vi "Control Panel Sensors.vi"(11 "Control Panel Motors":T2) -> (1 "Color":T1, 2 "Arm Out":bool, 3 "Arm In":bool, 4 "Control Panel Full":dbl, 6 "Control Panel":dbl(knob) scale=0.0..1.0, 8 "Arm":dbl(knob) scale=0.0..1.0)   [LabVIEW 2019]
uses:
  Control Panel Motors.ctl
  Color.ctl
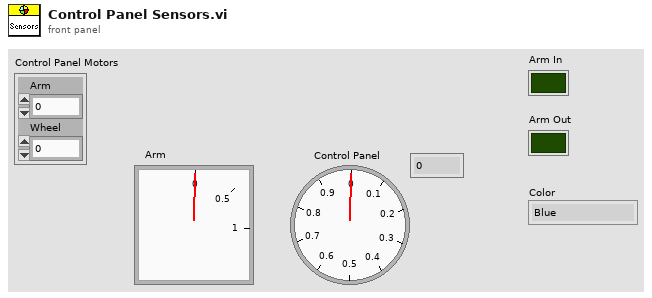
[diagram p1: front panel]
types:
  T1 = typedef "Color.ctl" = enum16{"Blue", "Green", "Red", "Yellow"}
  T2 = typedef "Control Panel Motors.ctl" = cluster{"Arm":dbl, "Wheel":dbl}
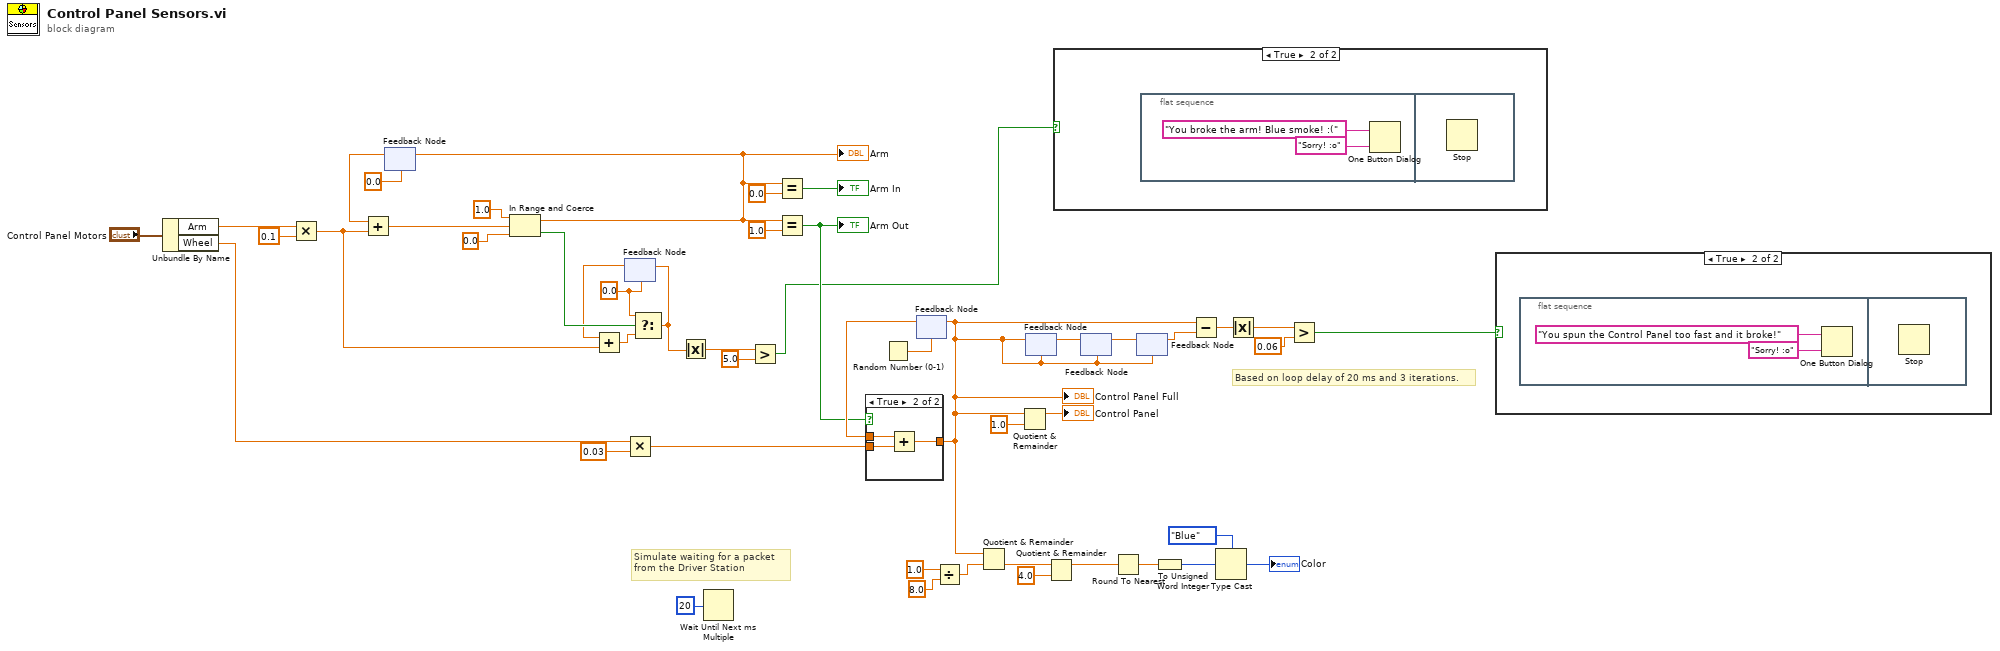
[diagram p0: block diagram]
diagram:
  w16 = 0.0
  # "Based on loop delay of 20 ms and 3 iterations."
  # "Simulate waiting for a packet \nfrom the Driver Station"
  n1 = Unbundle By Name("Control Panel Motors") -> ("Arm"=w34:dbl, "Wheel"=w37:dbl)
  n2 = Multiply(x=w34, y=0.1) -> (x*y=w13:dbl)
  n3 = feedback #1(0.0) -> (w33:dbl)
  n4 = Add(x=w33, y=w13) -> (x+y=w18:dbl)
  n5 = In Range and Coerce(upper limit=1.0, x=w18, lower limit=0.0) -> (coerced(x)=w22:dbl, In Range?=w17:bool)
  "Arm" <- w22
  n6 = feedback-in #1(w22) -> ()
  n7 = feedback #2(w16) -> (w14:dbl)
  n8 = Add(x=w14, y=w13) -> (x+y=w15:dbl)
  n9 = Multiply(x=w37, y=0.03) -> (x*y=w44:dbl)
  n10 = Select(t=w16, s=w17, f=w15) -> (s? t:f=w12:dbl)
  n11 = feedback-in #2(w12) -> ()
  n12 = Absolute Value(x=w12) -> (abs(x)=w10:dbl)
  n13 = Wait Until Next ms Multiple(millisecond multiple=u32 20) -> ()  [unwired: 1 out]
  n14 = Greater?(x=w10, y=5.0) -> (0:w9:bool)
  n15 = Equal?(x=w22, y=0.0) -> (x = y?=→"Arm In":bool)
  n16 = Equal?(x=w22, y=1.0) -> (x = y?=w23:bool)
  "Arm Out" <- w23
  n17 = Random Number (0-1)() -> (number: 0 to 1=w47:dbl)
  n18 = feedback #3(w47) -> (w45:dbl)
  n19 = case shown="True" w23 {
    tunnel: w45 -> [w49 w52]
    tunnel: w44 -> [_ w51]
    tunnel: [w49 w50] -> w6
    frame False {
    }
    frame True {
      n20 = Add(x=w52, y=w51) -> (x+y=w50:dbl)
    }
  }
  "Control Panel Full" <- w6
  n21 = feedback-in #3(w6) -> ()
  n22 = Divide(x=1.0, y=8.0) -> (x/y=w29:dbl)
  n23 = Quotient & Remainder(x=w6, y=w29) -> (floor(x/y)=w26:dbl)  [unwired: 1 out]
  n24 = Quotient & Remainder(x=w6, y=1.0) -> (x-y*floor(x/y)=→"Control Panel":dbl)  [unwired: 1 out]
  n25 = feedback-in #4(w6) -> ()
  n26 = feedback #4(w6) -> (w8:dbl)
  n27 = Quotient & Remainder(x=w26, y=4.0) -> (x-y*floor(x/y)=w24:dbl)  [unwired: 1 out]
  n28 = case shown="True" w9 {
    frame False {
    }
    frame True {
      n29 = flat-sequence {
        frame #0 {
          n30 = One Button Dialog(message="You broke the arm! Blue smoke! :(", button name ("OK")="Sorry! :o") -> ()  [unwired: 1 out]
        }
        frame #1 {
          n31 = Stop() -> ()  [unwired: 1 in]
        }
      }
    }
  }
  n32 = feedback #5(w6) -> (w7:dbl)
  n33 = feedback-in #5(w8) -> ()
  n34 = Round To Nearest(number=w24) -> (nearest integer value=w41:dbl)
  n35 = feedback #6(w6) -> (w5:dbl)
  n36 = feedback-in #6(w7) -> ()
  n37 = To Unsigned Word Integer(number=w41) -> (unsigned 16bit integer=w40:u16)
  n38 = Subtract(x=w6, y=w5) -> (x-y=w4:dbl)
  n39 = Type Cast(type=Color."Blue" ("Color"), x=w40) -> (*(type *) &x=→"Color":T1)
  n40 = Absolute Value(x=w4) -> (abs(x)=w3:dbl)
  n41 = Greater?(x=w3, y=0.06) -> (0:w1:bool)
  n42 = case shown="True" w1 {
    frame False {
    }
    frame True {
      n43 = flat-sequence {
        frame #0 {
          n44 = One Button Dialog(message="You spun the Control Panel too fast and it broke!", button name ("OK")="Sorry! :o") -> ()  [unwired: 1 out]
        }
        frame #1 {
          n45 = Stop() -> ()  [unwired: 1 in]
        }
      }
    }
  }
